vi "CreateActionQueues.vi"(8 "Error In":errorcluster) -> (0 "Error Out":errorcluster, 3 "Action Queues":T1)   [LabVIEW 2012]
uses:
  ActionQueues.ctl
  UIActionQueueElement.ctl
  UIAction.ctl
  HardwareActionQueueElement.ctl
  HardwareAction.ctl
  HeaterActionQueueElement.ctl
  HeaterAction.ctl
  MFCActionQueueElement.ctl
  MFCAction.ctl
  LogActionQueueElement.ctl
  LogAction.ctl
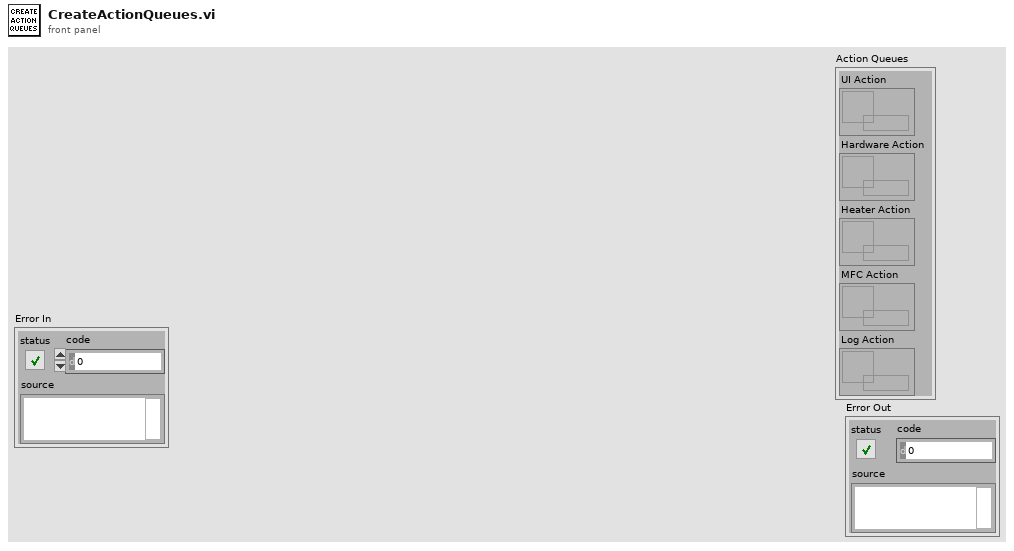
[diagram p1: front panel]
types:
  T1 = typedef "ActionQueues.ctl" = cluster{"UI Action":refnum<queue>, "Hardware Action":refnum<queue>, "Heater Action":refnum<queue>, "MFC Action":refnum<queue>, "Log Action":refnum<queue>}
  T2 = typedef "HeaterActionQueueElement.ctl" = cluster{"Action":T3, "Data":variant}
  T3 = typedef "HeaterAction.ctl" = enum16{"Initialize", "Start", "Read", "Write", "Stop", "Error", "Shutdown"}
  T4 = typedef "MFCActionQueueElement.ctl" = cluster{"Action":T5, "Data":variant}
  T5 = typedef "MFCAction.ctl" = enum16{"Initialize", "Start", "Read", "Write", "Stop", "Error", "Shutdown"}
  T6 = typedef "HardwareActionQueueElement.ctl" = cluster{"Action":T7, "Data":variant}
  T7 = typedef "HardwareAction.ctl" = enum16{"Initialize", "Collect", "Shutdown"}
  T8 = typedef "LogActionQueueElement.ctl" = cluster{"Action":T9, "Data":variant}
  T9 = typedef "LogAction.ctl" = enum16{"Initialize", "Start", "Log", "Stop", "Error", "Shutdown"}
  T10 = typedef "UIActionQueueElement.ctl" = cluster{"Action":T11, "Data":variant}
  T11 = typedef "UIAction.ctl" = enum16{"Initialize", "Connect", "MFC Connected", "Heater Connected", "Disconnect", "MFC Disconnected", "Heater Disconnected", "Configure MFC", "Configure Heater", "Open Log", "Close Log", "Shutdown"}
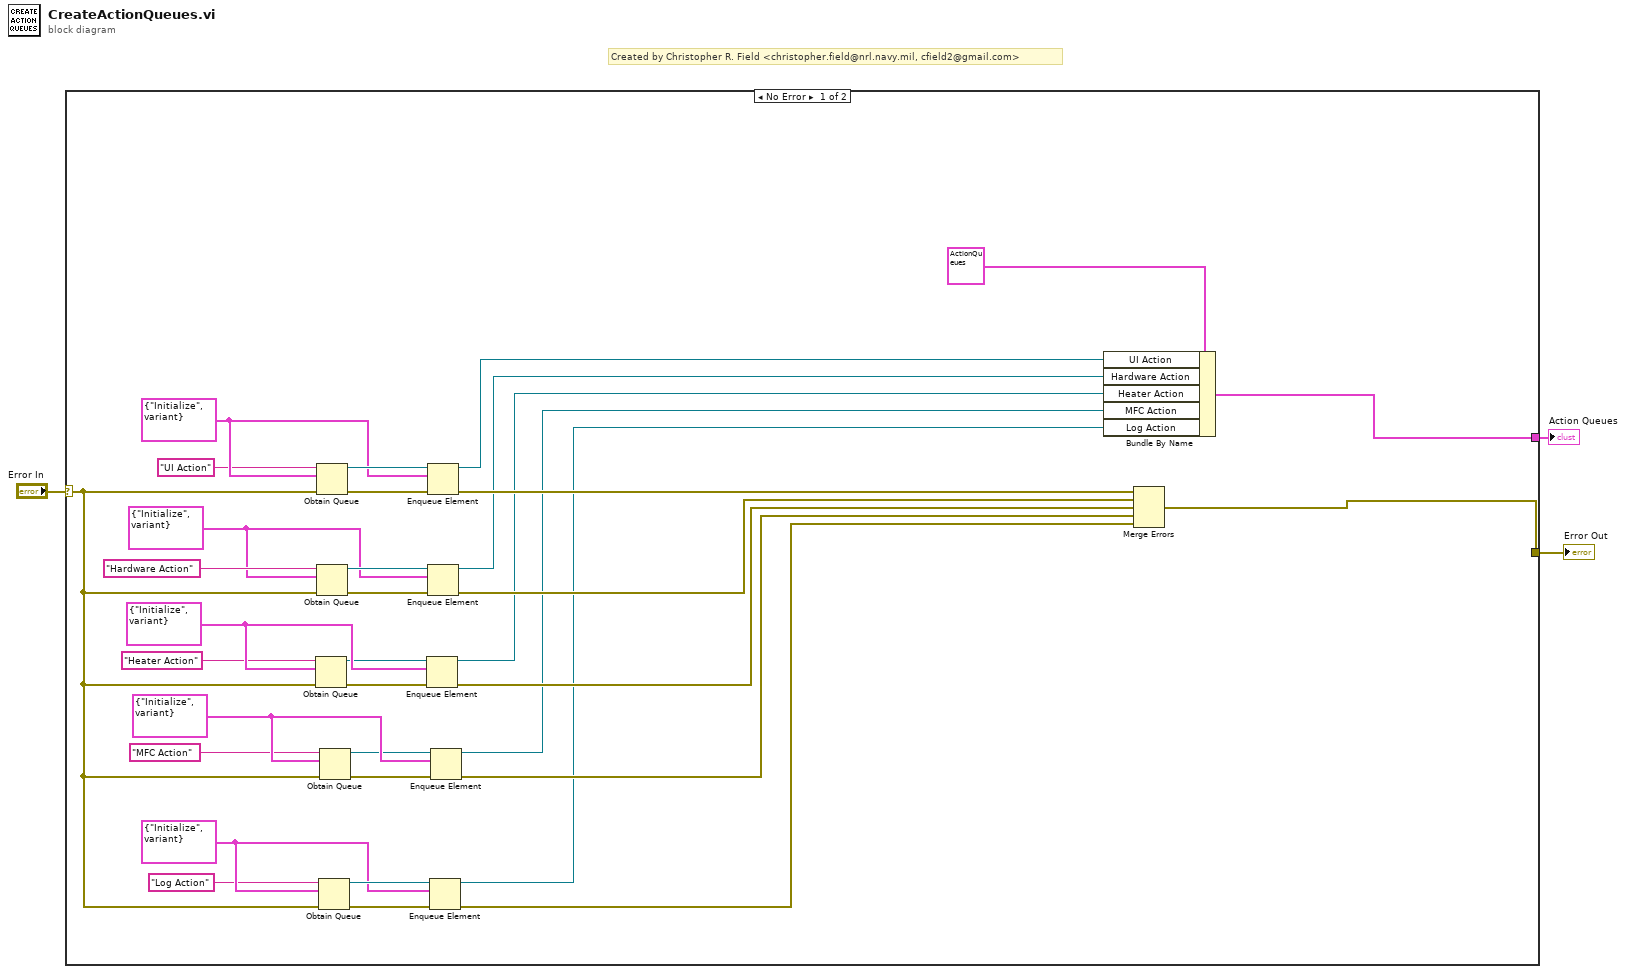
[diagram p0: block diagram]
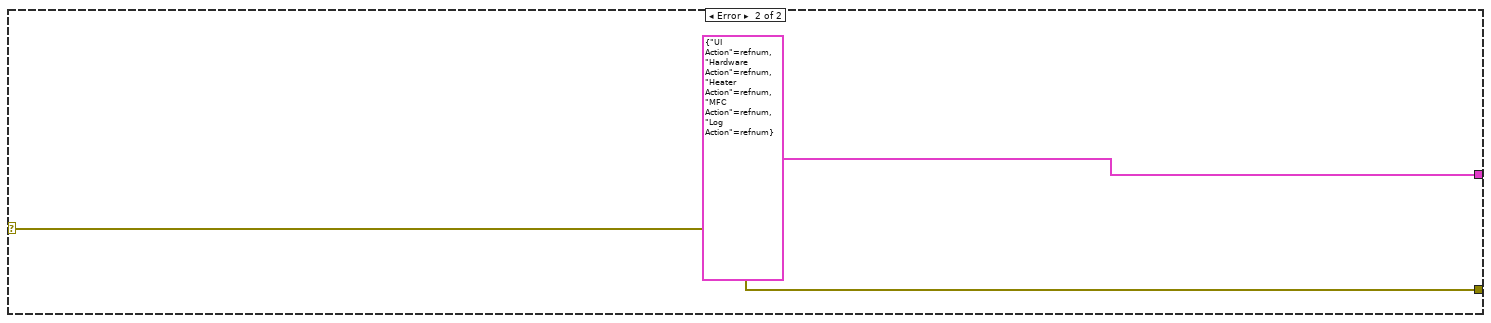
[diagram p2: hidden frame]
diagram:
  # "Created by Christopher R. Field <christopher.field@nrl.navy.mil, cfield2@gmail.com>"
  n1 = case shown="No Error" "Error In" {
    selector: "Error In" -> [w11 w39]
    tunnel: [w31 T1 {"UI Action"=refnum, "Hardware Action"=refnum, "Heater Action"=refnum, "MFC Action"=refnum, "Log Action"=refnum} ("Action Queues")] -> w2
    tunnel: [w29 w39] -> w1
    frame No Error {
      w19 = T2 {"Action"=enum."Initialize", "Data"=variant} ("Heater Action Queue Element")
      w15 = T4 {"Action"=enum."Initialize", "Data"=variant} ("MFC Action Queue Element")
      w21 = T6 {"Action"=enum."Initialize", "Data"=variant} ("Hardware Action Queue Element")
      w23 = T8 {"Action"=enum."Initialize", "Data"=variant} ("Log Action Queue Element")
      w35 = T10 {"Action"=enum."Initialize", "Data"=variant} ("UI Action Queue Element")
      n2 = Obtain Queue(name (unnamed)="Heater Action", element data type=w19, error in (no error)=w11) -> (queue out=w18:refnum<queue>, error out=w17:errorcluster)  [unwired: 2 in, 1 out]
      n3 = Obtain Queue(name (unnamed)="UI Action", element data type=w35, error in (no error)=w11) -> (queue out=w37:refnum<queue>, error out=w36:errorcluster)  [unwired: 2 in, 1 out]
      n4 = Obtain Queue(name (unnamed)="Hardware Action", element data type=w21, error in (no error)=w11) -> (queue out=w28:refnum<queue>, error out=w27:errorcluster)  [unwired: 2 in, 1 out]
      n5 = Obtain Queue(name (unnamed)="Log Action", element data type=w23, error in (no error)=w11) -> (queue out=w25:refnum<queue>, error out=w24:errorcluster)  [unwired: 2 in, 1 out]
      n6 = Obtain Queue(name (unnamed)="MFC Action", element data type=w15, error in (no error)=w11) -> (queue out=w14:refnum<queue>, error out=w13:errorcluster)  [unwired: 2 in, 1 out]
      n7 = Enqueue Element(queue=w18, element=w19, error in (no error)=w17) -> (queue out=w6:refnum<queue>, error out=w9:errorcluster)  [unwired: 1 in, 1 out]
      n8 = Enqueue Element(queue=w37, element=w35, error in (no error)=w36) -> (queue out=w32:refnum<queue>, error out=w30:errorcluster)  [unwired: 1 in, 1 out]
      n9 = Enqueue Element(queue=w28, element=w21, error in (no error)=w27) -> (queue out=w20:refnum<queue>, error out=w10:errorcluster)  [unwired: 1 in, 1 out]
      n10 = Enqueue Element(queue=w25, element=w23, error in (no error)=w24) -> (queue out=w4:refnum<queue>, error out=w7:errorcluster)  [unwired: 1 in, 1 out]
      n11 = Enqueue Element(queue=w14, element=w15, error in (no error)=w13) -> (queue out=w5:refnum<queue>, error out=w8:errorcluster)  [unwired: 1 in, 1 out]
      n12 = Bundle By Name(cluster=T1 {"UI Action"=refnum, "Hardware Action"=refnum, "Heater Action"=refnum, "MFC Action"=refnum, "Log Action"=refnum} ("Action Queues"), "UI Action"=w32, "Hardware Action"=w20, "Heater Action"=w6, "MFC Action"=w5, "Log Action"=w4) -> (w31:T1)
      n13 = Merge Errors(w30, w10, w9, w8, w7) -> (w29:errorcluster)
    }
    frame Error {
    }
  }
  "Action Queues" <- w2
  "Error Out" <- w1
